vi "set window position.vi"(8 "Error In":errorcluster, 10 "Control VI":refnum<vi>, 11 "Left VI":refnum<vi>) -> (0 "Error Out":errorcluster)   [LabVIEW 2019]
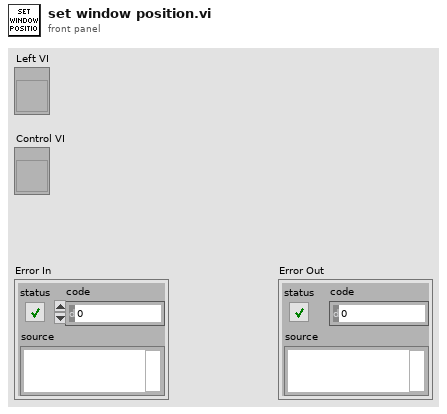
[diagram p1: front panel]
types:
  T1 = typedef "LVRectTypeDef.ctl" = cluster{"Left":i16, "Top":i16, "Right":i16, "Bottom":i16}
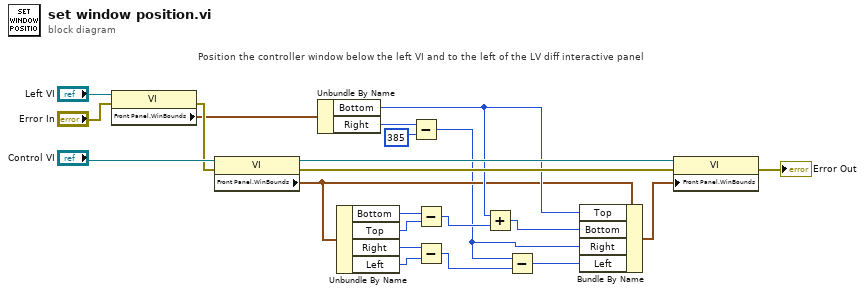
[diagram p0: block diagram]
diagram:
  # "Position the controller window below the left VI and to the left of the LV diff interactive panel"
  n1 = property class="VI"(reference="Left VI", error in="Error In") -> (error out=w19:errorcluster, "Front Panel.WinBounds"=w5:T1)  [unwired: 1 out]
  n2 = property class="VI"(reference="Control VI", error in=w19) -> (reference out=w17:refnum<vi>, error out=w18:errorcluster, "Front Panel.WinBounds"=w6:T1)
  n3 = Unbundle By Name(w5) -> ("Bottom"=w11:i16, "Right"=w3:i16)
  n4 = Unbundle By Name(w6) -> ("Bottom"=w8:i16, "Top"=w9:i16, "Right"=w13:i16, "Left"=w14:i16)
  n5 = Subtract(x=w3, y=i16 385) -> (x-y=w2:i16)
  n6 = Subtract(x=w8, y=w9) -> (x-y=w10:i16)
  n7 = Subtract(x=w13, y=w14) -> (x-y=w15:i16)
  n8 = Add(x=w11, y=w10) -> (x+y=w12:i16)
  n9 = Subtract(x=w2, y=w15) -> (x-y=w16:i16)
  n10 = Bundle By Name(cluster=w6, "Top"=w11, "Bottom"=w12, "Right"=w2, "Left"=w16) -> (w7:T1)
  n11 = property class="VI"(reference=w17, error in=w18, "Front Panel.WinBounds"=w7) -> (error out=→"Error Out":errorcluster)  [unwired: 1 out]
